vi "select_type.vi"(8 "Error in (no error)":errorcluster, 10 "type":string, 11 "Connection In":refnum<k7>) -> (0 "Error out":errorcluster, 2 "nombre d'heures":string, 3 "Connection Out":refnum<k7>)   [LabVIEW 2019]
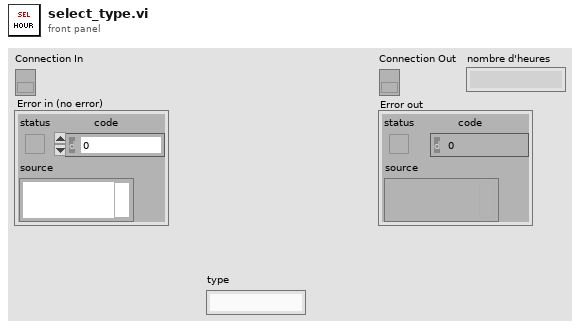
[diagram p1: front panel]
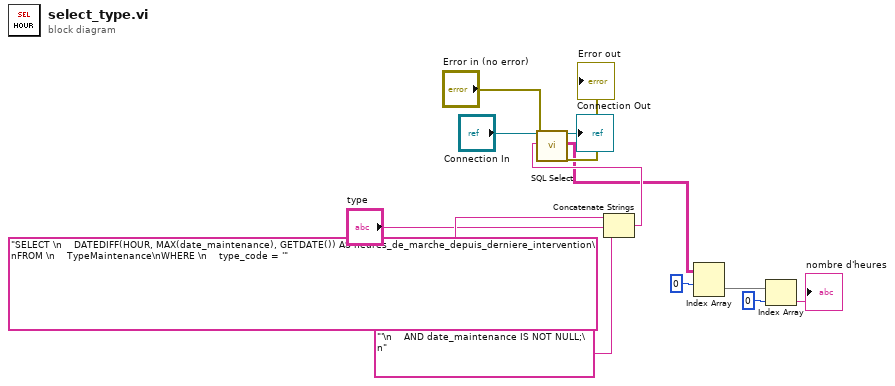
[diagram p0: block diagram]
diagram:
  n1 = Concatenate Strings("SELECT \n    DATEDIFF(HOUR, MAX(date_maintenance), GETDATE()) AS heures_de_marche_depuis_derniere_intervention\nFROM \n    TypeMaintenance\nWHERE \n    type_code = '" ("string"), "type", "'\n    AND date_maintenance IS NOT NULL;\n" ("string")) -> (w9:string)
  n2 = call <vilib>:"SQL Select.vi"("Connection In"="Connection In", "SQL Query"=w9, "Error in (no error)"="Error in (no error)") -> ("Connection Out"=→"Connection Out":refnum<k7>, "Data"=w2:string[][], "Error out"=→"Error out":errorcluster)  [unwired: 14 in]
  n3 = Index Array(array=w2, index (row)=0) -> (element=w3:string[])  [unwired: 1 in]
  n4 = Index Array(array=w3, index=0) -> (element=→"nombre d'heures":string)
